vi "Waveform array Read.vi"(4 "error in (no error)":errorcluster, 6 "Container State":T2, 7 "Display State In":T1) -> (0 "error out":errorcluster, 2 "Value":dbl[](array[numeric]), 3 "Display State Out":T1)   [LabVIEW 2012, in "Waveform Control.xctl"]
uses:
  Waveform Control.xctl
  <vilib>/_xctls/Container State.ctl
  Controls/State.ctl
  <vilib>/_xctls/XControlSupport.lvlib
panel:
  # "Replace the Value Indicator below with an Indicator of desired type.\nDo not remove this Indicator or the others from the connector pane. \nDo not change the connector pane pattern.\nThe Value Indicator should always be the second terminal from top on the output side in the connector pane."
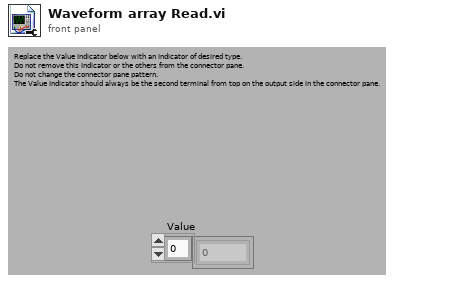
[diagram p1: front panel]
types:
  T1 = typedef "Waveform Control.xctl/State.ctl" = cluster{"Name":string}
  T2 = typedef "XControlSupport.lvlib/Container State.ctl" = cluster{"Indicator?":bool, "Run Mode?":bool, " Refnum":refnum<vi>}
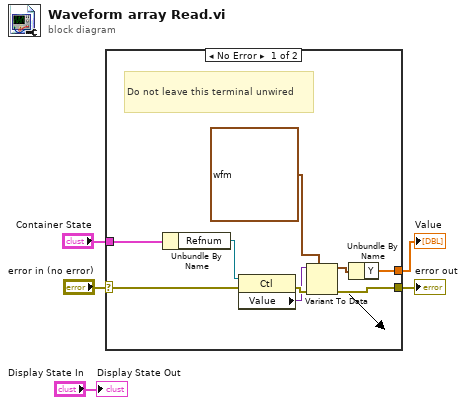
[diagram p0: block diagram]
diagram:
  n1 = case shown="No Error" "error in (no error)" {
    selector: "error in (no error)" -> [w7 w15]
    tunnel: "Container State" -> [w14 _]
    tunnel: [w8 _] -> w3
    tunnel: [w6 w15] -> w1
    frame No Error {
      # "Do not leave this terminal unwired"
      n2 = Unbundle By Name(w14) -> ("Refnum"=w13:refnum<vi>)
      n3 = property class="Ctl"(reference=w13, error in=w7) -> (error out=w12:errorcluster, "Value"=w11:variant)  [unwired: 1 out]
      n4 = Variant To Data(error in=w12, type=waveform(dbl) {"t0"=timestamp(0 s since 1904-01-01), "dt"=1.0, "Y"=[]} ("waveform"), Variant=w11) -> (data=w9:waveform(dbl), error out=w6:errorcluster)
      n5 = Unbundle By Name(w9) -> ("Y"=w8:dbl[])
    }
    frame Error {
    }
  }
  "error out" <- w1
  "Value" <- w3
  "Display State Out" <- "Display State In"
